vi "Parse metadata property names and values.vi"(0 "Data intput []":string[](array[string]), 1 "property names []":string[](array[string]), 3 "List param":bool, 5 "error in (no error)":errorcluster) -> (14 "Param list":string, 15 "Array":string[](array[string]), 16 "output cluster":T1, 19 "error out":errorcluster)   [LabVIEW 2019, in "metadata.lvclass"]
uses:
  metadata.lvclass
  Metadata output --cluster.ctl
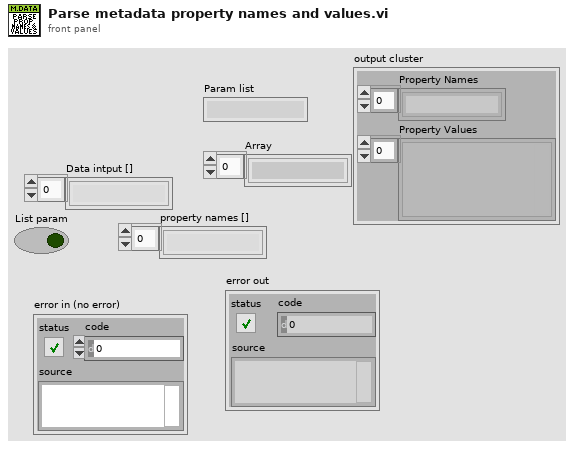
[diagram p1: front panel]
types:
  T1 = typedef "metadata.lvclass/Metadata output --cluster.ctl" = cluster{"Property Names":string[], "Property Values":variant[]}
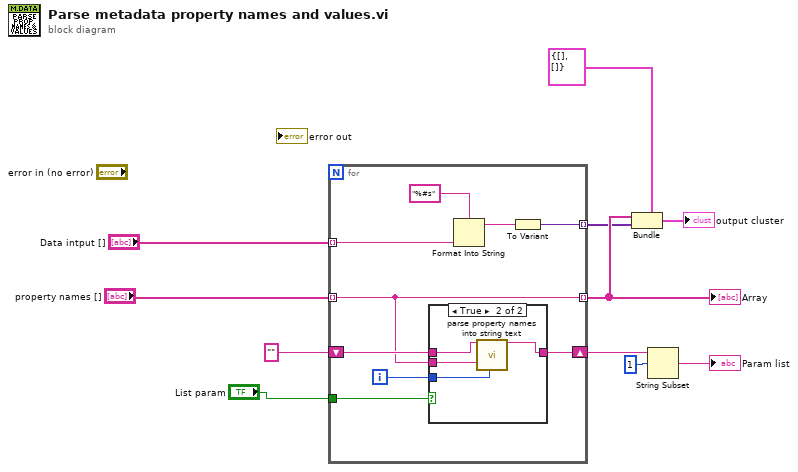
[diagram p0: block diagram]
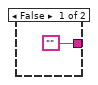
[diagram p2: hidden frame]
diagram:
  n1 = for {
    tunnel: [w15] -> w7 mode=indexing
    tunnel: "property names []" -> [w15] mode=indexing
    tunnel: [w19] -> w6 mode=indexing
    shift-right: [w14] -> w9
    shift-left: "" -> [w17]
    tunnel: "Data intput []" -> [w16] mode=indexing
    tunnel: "List param" -> [w12]
    i -> [w13]
    n2 = case shown="True" w12 {
      tunnel: w17 -> [_ w23]
      tunnel: w15 -> [_ w25]
      tunnel: ["" w22] -> w14
      tunnel: w13 -> [_ w24]
      frame False {
      }
      frame True {
        n3 = call "parse property names into string text.vi"("String in"=w23, "Property names"=w25, "Counter"=w24) -> ("String out"=w22:string)  [unwired: 15 in, 1 out]
      }
    }
    n4 = Format Into String(format string="%#s", w16) -> (resulting string=w20:string)  [unwired: 2 in, 1 out]
    n5 = To Variant(anything=w20) -> (Variant=w19:variant)
  }
  "Array" <- w7
  n6 = Bundle(cluster=T1 {"Property Names"=[], "Property Values"=[]} ("Metadata"), "Property Names"=w7, "Property Values"=w6) -> (→"output cluster":T1)
  n7 = String Subset(string=w9, offset (0)=1) -> (substring=→"Param list":string)  [unwired: 1 in]
